vi "Power Accuracy Retrieve Key Array for  Config.vi"(8 "error in (no error)":errorcluster, 9 "Datasheets":T10, 10 "Key Array In":T11, 11 "Connection Refnum":T1) -> (0 "error out":errorcluster, 2 "Power Accuracy Test Parameters":T2={"Stimulus"={"Power Start"=38, "Power Stop"=46, "Frequency Type"=enum."Band Edges", "Frequency Points"=[], "TX 1 Frequency (MHz)"={"Min"=0.0, "Max"=0.0}, "TX 2 Frequency (MHz)"={"Min"=0.0, "Max"=0.0}, "RX Frequency (MHz)"={"Min"=0.0, "Max"=0.0}, "Pad Model Number"="", "Pad Serial Number"="", "Pad Values"=[]}, "Measurement"={"DUT Port"=enum."Port 1", "Direction"=0}, "Display"={"Power"={"Min"=0, "Max"=0}, "Tolerance"={"Min"=0.0, "Max"=0.0}}, "Limit"={"Tolerance"=0.35}, "Calibration"={"Calibrated?"=FALSE}} {"Measurement"."Direction" items=["Reverse", "Forward", "Auxiliary"]}, 3 "Connection Refnum":T1)   [LabVIEW 2011]
uses:
  ITK EXT/utils/keyedarr.llb/Keyed Array.ctl
  Test Datasheets.ctl
  TypeDefs/Power Accuracy Test Parameters.ctl
  TypeDefs/Power Accuracy Stimulus Parameters.ctl
  TypeDefs/Power Accuracy Measurement Parameters.ctl
  BPIMCore EXT/HW IO/DUTport.ctl
  BPIMCore EXT/HW IO/MeasMode.ctl
  TypeDefs/Power Accuracy Display Parameters.ctl
  TypeDefs/Power Accuracy Limit Parameters.ctl
  TypeDefs/Power Accuracy Calibration State.ctl
  Summitek EXT/ODBC/SQL Controls/Connection Refnum.ctl
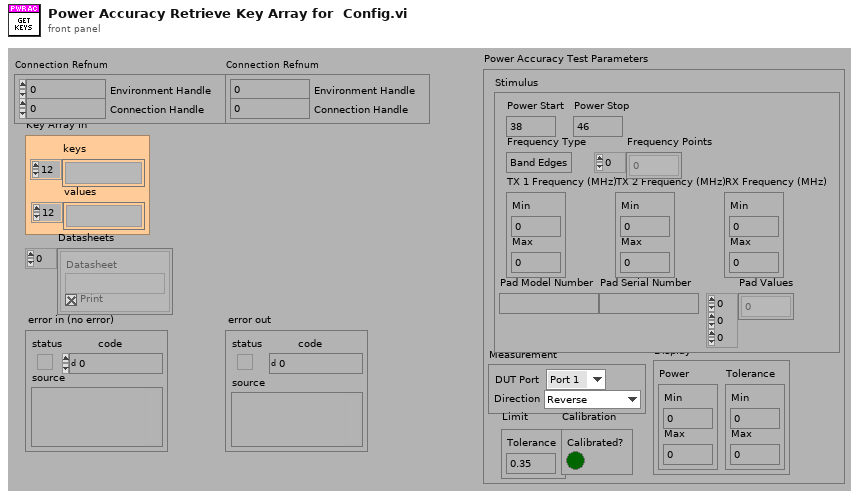
[diagram p1: front panel]
types:
  T1 = typedef "Connection Refnum.ctl" = cluster{"Environment Handle":i32, "Connection Handle":i32}
  T2 = typedef "Power Accuracy Test Parameters.ctl" = cluster{"Stimulus":T3, "Measurement":T4, "Display":T7, "Limit":T8, "Calibration":T9}
  T3 = typedef "Power Accuracy Stimulus Parameters.ctl" = cluster{"Power Start":i32, "Power Stop":i32, "Frequency Type":enum16{"Band Edges", "Custom"}, "Frequency Points":dbl[], "TX 1 Frequency (MHz)":cluster{"Min":dbl, "Max":dbl}, "TX 2 Frequency (MHz)":cluster{"Min":dbl, "Max":dbl}, "RX Frequency (MHz)":cluster{"Min":dbl, "Max":dbl}, "Pad Model Number":string, "Pad Serial Number":string, "Pad Values":dbl[][][]}
  T4 = typedef "Power Accuracy Measurement Parameters.ctl" = cluster{"DUT Port":T5, "Direction":T6}
  T5 = typedef "DUTport.ctl" = enum16{"Port 1", "Port 2"}
  T6 = typedef "MeasMode.ctl" = u16
  T7 = typedef "Power Accuracy Display Parameters.ctl" = cluster{"Power":cluster{"Min":i32, "Max":i32}, "Tolerance":cluster{"Min":dbl, "Max":dbl}}
  T8 = typedef "Power Accuracy Limit Parameters.ctl" = cluster{"Tolerance":dbl}
  T9 = typedef "Power Accuracy Calibration State.ctl" = cluster{"Calibrated?":bool}
  T10 = typedef "Test Datasheets.ctl" = cluster{"Datasheet":string, "Print":bool}[]
  T11 = typedef "Keyed Array.ctl" = cluster{"keys":string[], "values":string[]}
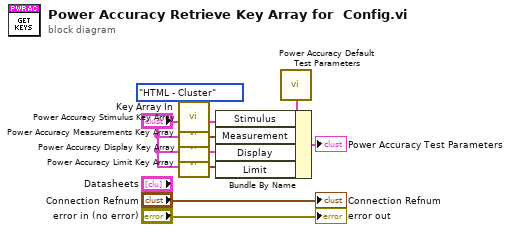
[diagram p0: block diagram]
diagram:
  w3 = enum16{"Cluster - HTML", "HTML - Cluster"}."HTML - Cluster" ("Conversion")
  n1 = call "Power Accuracy Stimulus Key Array.vi"("Conversion"=w3, "Stimulus Key Array In"="Key Array In") -> ("Stimulus Cluster Out"=w7:T3)  [unwired: 5 in, 1 out]
  n2 = call "Power Accuracy Measurements Key Array.vi"("Conversion"=w3, "Measurements Key Array In"="Key Array In") -> ("Measurements Cluster Out"=w6:T4)  [unwired: 5 in, 1 out]
  n3 = call "Power Accuracy Display Key Array.vi"("Conversion"=w3, "Display Key Array In"="Key Array In") -> ("Display Cluster Out"=w5:T7)  [unwired: 5 in, 1 out]
  n4 = call "Power Accuracy Limit Key Array.vi"("Conversion"=w3, "Limits Key Array In"="Key Array In") -> ("Limits Cluster Out"=w4:T8)  [unwired: 5 in, 1 out]
  n5 = call "Power Accuracy Default Test Parameters.vi"() -> ("Default Power Accuracy Test Parameters"=w8:T2)
  n6 = Bundle By Name(cluster=w8, "Stimulus"=w7, "Measurement"=w6, "Display"=w5, "Limit"=w4) -> (→"Power Accuracy Test Parameters":T2)
  "error out" <- "error in (no error)"
  "Connection Refnum" <- "Connection Refnum"
